vi "GetType.vi"(8 "error in (no error)":errorcluster, 11 "Update_Referenced Msg":refnum<class "Update_Referenced Msg.lvclass">) -> (0 "error out":errorcluster, 2 "Data Sample":variant, 3 "Update_Referenced Msg":refnum<class "Update_Referenced Msg.lvclass">)   [LabVIEW 2015, in "CS++Motor.lvlib" / "Update_Referenced Msg.lvclass"]
uses:
  Update_Referenced Msg.lvclass
  Update_Referenced Msg.lvclass/Update_Referenced Msg.ctl
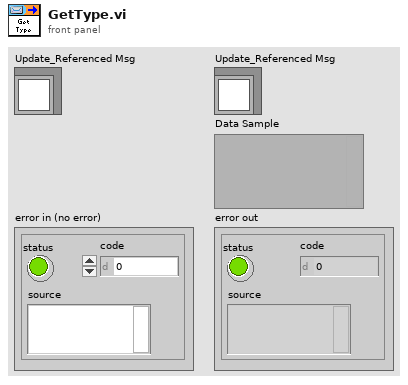
[diagram p1: front panel]
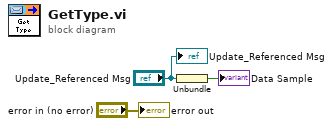
[diagram p0: block diagram]
diagram:
  n1 = Unbundle("Update_Referenced Msg") -> (→"Data Sample":bool)
  "error out" <- "error in (no error)"
  "Update_Referenced Msg" <- "Update_Referenced Msg"
